vi "MonitorAccelerometer.vi"(11 "Settings":T1={"Channel0FIFO"="Accel1Channel0FIFO", "Channel1FIFO"="Accel1Channel1FIFO", "Channel2FIFO"="Accel1Channel2FIFO", "StartSignal"="Accel/Start", "StopSignal"="Accel/Stop", "Channel0Signal"="Accel/AI0", "Channel1Signal"="Accel/AI1", "Channel2Signal"="Accel/AI2", "SampleTrigger"="Sync/Trig0", "TimestampFIFO"="Accel1TimestampFIFO", "TimestampRegister"="TimestampRegister"}) -> ()   [LabVIEW 2016, in "FPGAMonitorAccelerometer.lvlib"]
uses:
  FPGAMonitorAccelerometer.lvlib
  DataTypes/MonitorAccelerometerSettings.ctl
  <vilib>/rvi/Emulation/niFpgaGetClockAttributes.vi
  <vilib>/rvi/Emulation/niFpgaSctlEmulationGetInTimedLoop.vi
  <vilib>/rvi/Emulation/niFpgaEmulationReportErrorSimple.vi
  <vilib>/rvi/eio/common/nirviEmuTemplateMethod_errors.vi
  <vilib>/rvi/DataTransferAndStorage/Container/Common/niFpgaContainerExecOnDevCompGetState.vi
  <vilib>/rvi/Emulation/niFpgaEmulationIsFPGAContextNoSignature.vi
  <vilib>/rvi/DataTransferAndStorage/Container/Common/niFpgaContainerGetUniqueNameForEmu.vi
  <vilib>/rvi/Memory/Memory_Emulation/niFpgaMemoryEmulationCacheClearOnFirstRun.vi
  <vilib>/rvi/Memory/Memory_Emulation/nirvimemoryEmulationManagerCache_MakeExclusive.vi
  <vilib>/rvi/Memory/Memory_Emulation/niFpgaMemoryEmulationValidateCache.vi
  <vilib>/rvi/Memory/Memory_Emulation/nirvimemoryEmulationManagerCache_InsertValue.vi
  <vilib>/Utility/error.llb/Clear Errors.vi
  <vilib>/rvi/Memory/Memory_Emulation/nirvimemoryEmulationManagerCache_ReleaseExclusive.vi
  <vilib>/rvi/Memory/Memory_Emulation/nirvimemoryEmulationManagerCache_GetValue.vi
  <vilib>/rvi/Memory/Memory_Emulation/nirvimemoryEmulationManagerCache_SetValue.vi
  <vilib>/rvi/Emulation/niFpgaProcessEmulError.vi
  <vilib>/rvi/errors/niFpgaSetErrorForExecOnDevCompSimple.vi
  <vilib>/rvi/eio/common/nirviEmuReportErrorAndStop.vi
  <vilib>/rvi/FIFO/Fifo_Resource/nirvififoEmulationSetSize.vi
  <vilib>/rvi/FIFO/Fifo_Resource/nirviFifoEmulationQueueMgr.vi
  <instcachedir>/0/nirviFifoEmulationQueueMgr_E5CAEC123FF24DC58D834DCA3CDAA9B5.lvgen/nirviFifoEmulationQueueMgr_E5CAEC123FF24DC58D834DCA3CDAA9B5_007.vi
  <vilib>/rvi/FIFO/Fifo_Resource/nirvififoEmulationDetermineInputValidOut.vi
  <vilib>/rvi/FIFO/Fifo_Resource/nirvififoEmulationCreateLock.vi
  <vilib>/rvi/FIFO/Fifo_Resource/nirvififoEmulationObtainLock.vi
  <vilib>/rvi/FIFO/Fifo_Resource/nirvififoEmulationReleaseLock.vi
  <vilib>/rvi/occurrence/nirviWaitOnOccurrenceBase.vi
  <vilib>/rvi/errors/nirviReportUnexpectedCaseInternalError.vi
  <vilib>/rvi/errors/nirviReportUnexpectedCaseInternalError (U32).vi
  <vilib>/rvi/interface/RandomDataEmulation/niFpgaRandomDataHandleErrors.vi
  <instcachedir>/0/nirviFifoEmulationQueueMgr_E5CAEC123FF24DC58D834DCA3CDAA9B5.lvgen/nirviFifoEmulationQueueMgr_E5CAEC123FF24DC58D834DCA3CDAA9B5_005.vi
  <vilib>/rvi/Emulation/niFpgaCriticalErrorInLSC.vi
  <vilib>/eio/EIOMethodNode/EIOMethodNode.xnode
  <vilib>/rvi/DataTransferAndStorage/Container/XNode/niFpgaContainer.xnode
  <vilib>/rvi/DataTransferAndStorage/Register/Emulation/niFpgaRegisterEmulationRefIn.vi
  <vilib>/rvi/FIFO/Fifo_Resource/niFpgaFifoEmulationRefIn.vi
  <vilib>/eio/EIONode/EIONode.xnode
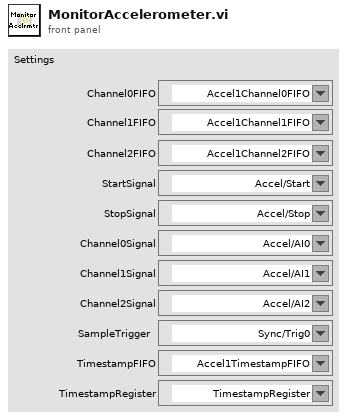
[diagram p1: front panel]
types:
  T1 = typedef "FPGAMonitorAccelerometer.lvlib/MonitorAccelerometerSettings.ctl" = cluster{"Channel0FIFO":refnum<k21>, "Channel1FIFO":refnum<k21>, "Channel2FIFO":refnum<k21>, "StartSignal":refnum<k21>, "StopSignal":refnum<k21>, "Channel0Signal":refnum<k21>, "Channel1Signal":refnum<k21>, "Channel2Signal":refnum<k21>, "SampleTrigger":refnum<k21>, "TimestampFIFO":refnum<k21>, "TimestampRegister":refnum<k21>}
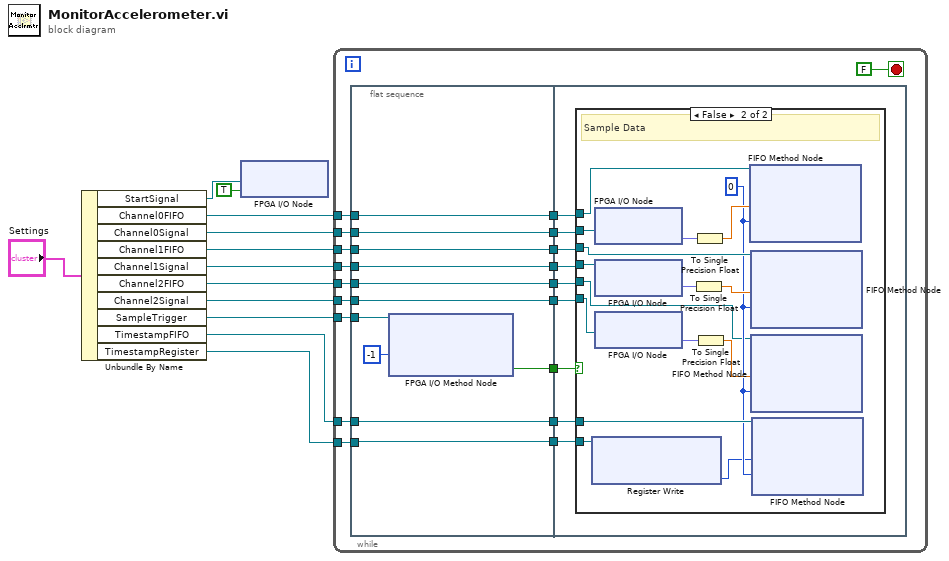
[diagram p0: block diagram]
diagram:
  n1 = Unbundle By Name("Settings") -> ("StartSignal"=w3:refnum<k21>, "Channel0FIFO"=w11:refnum<k21>, "Channel0Signal"=w10:refnum<k21>, "Channel1FIFO"=w9:refnum<k21>, "Channel1Signal"=w8:refnum<k21>, "Channel2FIFO"=w7:refnum<k21>, "Channel2Signal"=w6:refnum<k21>, "SampleTrigger"=w5:refnum<k21>, "TimestampFIFO"=w2:refnum<k21>, "TimestampRegister"=w1:refnum<k21>)
  n2 = xnode "FPGA I/O Node"("I/O Item"=TRUE, "FPGA I/O In"=w3) -> ()  [unwired: 1 out]
  n3 = while {
    tunnel: w11 -> [w24]
    tunnel: w10 -> [w25]
    tunnel: w9 -> [w26]
    tunnel: w8 -> [w27]
    tunnel: w7 -> [w28]
    tunnel: w6 -> [w29]
    tunnel: w5 -> [w30]
    tunnel: w2 -> [w16]
    tunnel: w1 -> [w13]
    stop <- FALSE stop-if-true
    n4 = flat-sequence {
      tunnel: w30 -> [w42]
      tunnel: w29 -> [w41]
      tunnel: w28 -> [w40]
      tunnel: w27 -> [w39]
      tunnel: w26 -> [w38]
      tunnel: w25 -> [w37]
      tunnel: w24 -> [w36]
      tunnel: [w41] -> w23
      tunnel: [w40] -> w22
      tunnel: [w39] -> w21
      tunnel: [w38] -> w20
      tunnel: [w37] -> w19
      tunnel: [w36] -> w18
      tunnel: [w35] -> w17
      tunnel: w16 -> [w34]
      tunnel: [w34] -> w15
      tunnel: [w33] -> w14
      tunnel: w13 -> [w33]
      tunnel: w23 -> [w46]
      tunnel: w22 -> [w47]
      tunnel: w21 -> [w48]
      tunnel: w20 -> [w49]
      tunnel: w19 -> [w50]
      tunnel: w18 -> [w51]
      tunnel: w17 -> [w43]
      tunnel: w15 -> [w45]
      tunnel: w14 -> [w44]
      frame #0 {
        n5 = xnode "FPGA I/O Method Node"("FPGA I/O In"=w42, "Timeout"=-1) -> ("Timed Out"=w35:bool)  [unwired: 1 out]
      }
      frame #1 {
        n6 = case shown="False" w43 {
          tunnel: w50 -> [_ w62]
          tunnel: w51 -> [_ w63]
          tunnel: w49 -> [_ w59]
          tunnel: w48 -> [_ w58]
          tunnel: w47 -> [_ w52]
          tunnel: w46 -> [_ w61]
          tunnel: w45 -> [_ w56]
          tunnel: w44 -> [_ w54]
          frame True {
            # "Dont Sample Data"
          }
          frame False {
            w55 = 0 ("Timeout")
            # "Sample Data"
            n7 = xnode "Register Write"("Register In"=w54) -> ("Data"=w53:u64)  [unwired: 1 out]
            n8 = xnode "FPGA I/O Node"("FPGA I/O In"=w62) -> ("I/O Item"=w67:fxp<+/-,24,7>)  [unwired: 1 out]
            n9 = xnode "FPGA I/O Node"("FPGA I/O In"=w58) -> ("I/O Item"=w66:fxp<+/-,24,7>)  [unwired: 1 out]
            n10 = xnode "FPGA I/O Node"("FPGA I/O In"=w61) -> ("I/O Item"=w65:fxp<+/-,24,7>)  [unwired: 1 out]
            n11 = To Single Precision Float(number=w66) -> (single precision float=w57:sgl)
            n12 = To Single Precision Float(number=w67) -> (single precision float=w64:sgl)
            n13 = To Single Precision Float(number=w65) -> (single precision float=w60:sgl)
            n14 = xnode ("FIFO Method Node")("Element"=w64, "Timeout"=w55, "FIFO In"=w63) -> ()  [unwired: 2 out]
            n15 = xnode ("FIFO Method Node")("Element"=w57, "Timeout"=w55, "FIFO In"=w59) -> ()  [unwired: 2 out]
            n16 = xnode ("FIFO Method Node")("Element"=w60, "Timeout"=w55, "FIFO In"=w52) -> ()  [unwired: 2 out]
            n17 = xnode ("FIFO Method Node")("Element"=w53, "Timeout"=w55, "FIFO In"=w56) -> ()  [unwired: 2 out]
          }
        }
      }
    }
  }
